vi "test_fastcast.vi"() -> ()   [LabVIEW 2013]
panel:
  out "data string":string
  out "default string":string[](array[string])
  out "default type":u8[](array[numeric]) format="%.0x"
  out "OK":bool[][](array[boolean])
  out "result":variant[][](array[variant])
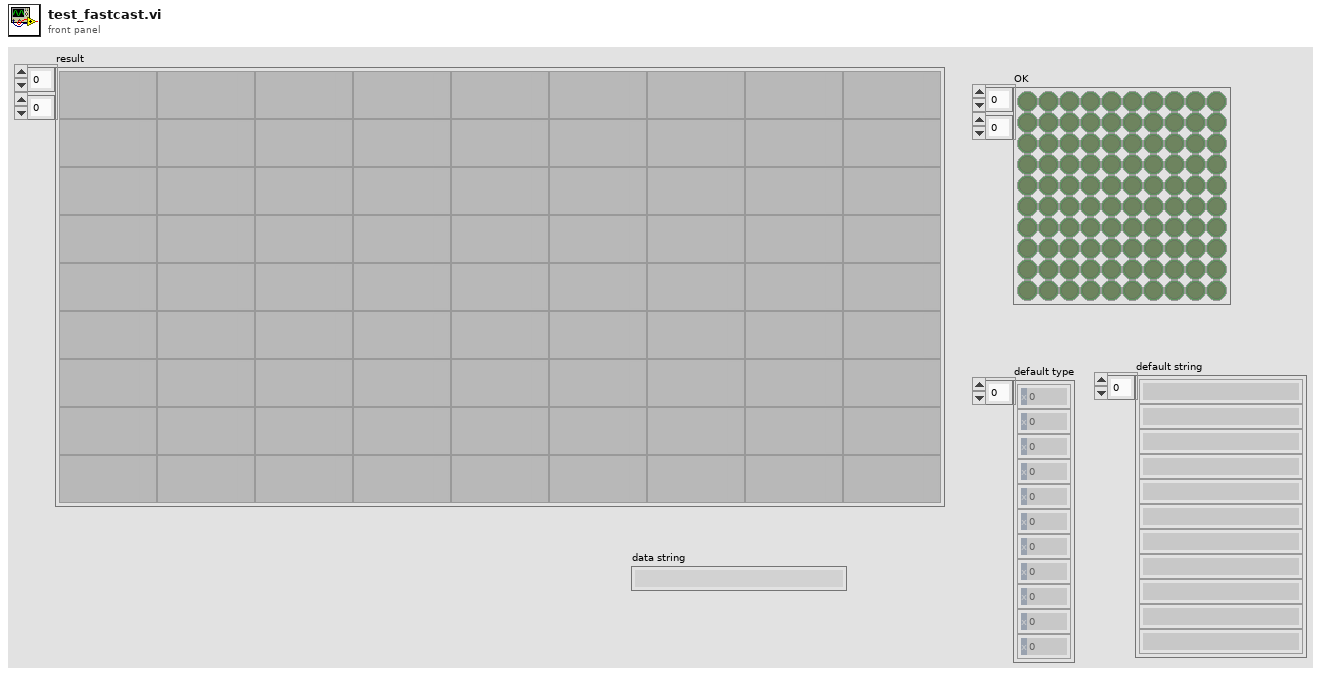
[diagram p1: front panel]
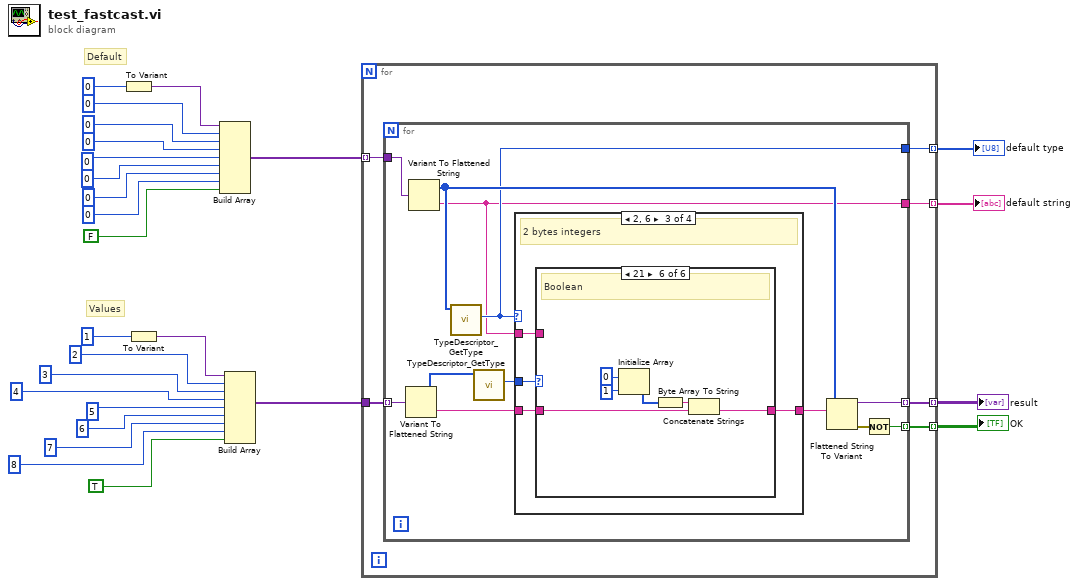
[diagram p0: block diagram]
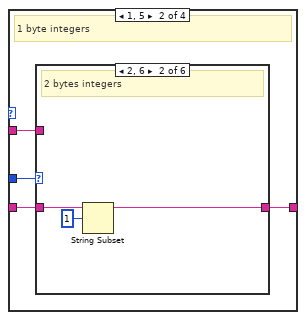
[diagram p3: hidden frame]
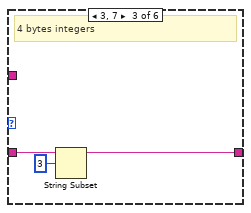
[diagram p5: hidden frame]
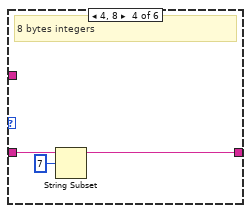
[diagram p6: hidden frame]
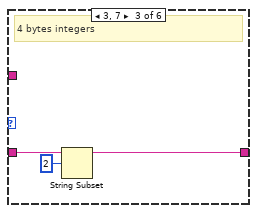
[diagram p11: hidden frame]
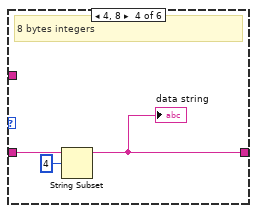
[diagram p12: hidden frame]
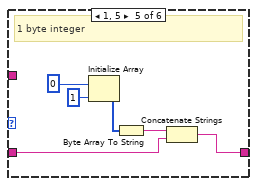
[diagram p13: hidden frame]
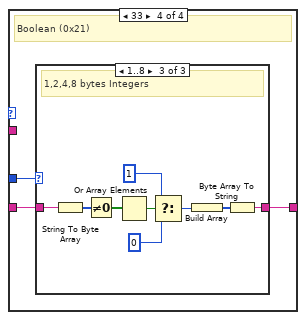
[diagram p14: hidden frame]
diagram:
  # "Values"
  # "Default"
  n1 = To Variant(anything=i8 0) -> (Variant=w25:variant)
  n2 = To Variant(anything=i8 1) -> (Variant=w2:variant)
  n3 = Build Array(w25, i16 0, 0, i64 0, u8 0, u16 0, u32 0, u64 0, FALSE) -> (w24:variant[])
  n4 = Build Array(w2, i16 2, 3, i64 4, u8 5, u16 6, u32 7, u64 8, TRUE) -> (w1:variant[])
  n5 = for {
    tunnel: w24 -> [w31] mode=indexing
    tunnel: w1 -> [w32]
    tunnel: [w30] -> w26 mode=indexing
    tunnel: [w29] -> w23 mode=indexing
    tunnel: [w28] -> w22 mode=indexing
    tunnel: [w27] -> w21 mode=indexing
    n6 = for {
      tunnel: w32 -> [w42] mode=indexing
      tunnel: w31 -> [w43]
      tunnel: [w41] -> w30 mode=indexing
      tunnel: [w44] -> w29 mode=indexing
      tunnel: [w34] -> w28
      tunnel: [w33] -> w27
      n7 = Variant To Flattened String(Variant=w42) -> (data string=w37:string, 1:w36:i16[])
      n8 = Variant To Flattened String(Variant=w43) -> (data string=w33:string, 1:w39:i16[])
      n9 = call "TypeDescriptor_GetType.vi"("type descriptor"=w39) -> ("Type"=w34:u8)  [unwired: 9 in, 1 out]
      n10 = call "TypeDescriptor_GetType.vi"("type descriptor"=w36) -> ("Type"=w35:u8)  [unwired: 9 in, 1 out]
      n11 = case shown="2, 6" w34 {
        tunnel: w37 -> [w45 w48 w63 w85]
        tunnel: [w45 w47 w62 w84] -> w38
        tunnel: w35 -> [_ w49 w64 w86]
        tunnel: w33 -> [_ w46 w61 _]
        frame Default {
        }
        frame 1, 5 {
          # "1 byte integers"
          n12 = case shown="2, 6" w49 {
            tunnel: w48 -> [_ w52 w55 w58 w59 w60]
            tunnel: [_ w50 w53 w56 w59 w60] -> w47
            tunnel: w46 -> [_ _ _ _ _ _]
            frame Default {
            }
            frame 2, 6 {
              # "2 bytes integers"
              n13 = String Subset(string=w52, offset (0)=1) -> (substring=w50:string)  [unwired: 1 in]
            }
            frame 3, 7 {
              # "4 bytes integers"
              n14 = String Subset(string=w55, offset (0)=3) -> (substring=w53:string)  [unwired: 1 in]
            }
            frame 4, 8 {
              # "8 bytes integers"
              n15 = String Subset(string=w58, offset (0)=7) -> (substring=w56:string)  [unwired: 1 in]
            }
            frame 1, 5 {
              # "1 bytesintegers"
            }
            frame 33 {
              # "Boolean"
            }
          }
        }
        frame 2, 6 {
          # "2 bytes integers"
          n16 = case shown="21" w64 {
            tunnel: w63 -> [_ w65 w68 w71 w73 w80]
            tunnel: [_ w65 w66 w69 w72 w79] -> w62
            tunnel: w61 -> [_ _ _ _ _ _]
            frame Default {
            }
            frame 2, 6 {
              # "2 bytes integers"
            }
            frame 3, 7 {
              # "4 bytes integers"
              n17 = String Subset(string=w68, offset (0)=2) -> (substring=w66:string)  [unwired: 1 in]
            }
            frame 4, 8 {
              # "8 bytes integers"
              n18 = String Subset(string=w71, offset (0)=4) -> (substring=w69:string)  [unwired: 1 in]
              "data string" <- w69
            }
            frame 1, 5 {
              # "1 byte integer"
              n19 = Initialize Array(u8 0, 1 ("dimension size")) -> (w75:u8[])
              n20 = Byte Array To String(unsigned byte array=w75) -> (string=w74:string)
              n21 = Concatenate Strings(w74, w73) -> (w72:string)
            }
            frame 33 {
              # "Boolean"
              n22 = Initialize Array(u8 0, 1 ("dimension size")) -> (w81:u8[])
              n23 = Byte Array To String(unsigned byte array=w81) -> (string=w78:string)
              n24 = Concatenate Strings(w78, w80) -> (w79:string)
            }
          }
        }
        frame 33 {
          # "Boolean (0x21)"
          n25 = case shown="1..8" w86 {
            tunnel: w85 -> [_ w87 w94]
            tunnel: [_ w87 w96] -> w84
            frame Default {
              # "Incompatible type"
            }
            frame 33 {
              # "Boolean (0x21)"
            }
            frame 1..8 {
              # "1,2,4,8 bytes Integers"
              n26 = String To Byte Array(string=w94) -> (unsigned byte array=w93:u8[])
              n27 = Not Equal To 0?(x=w93) -> (x != 0?=w92:bool[])
              n28 = Or Array Elements(Boolean array=w92) -> (logical OR=w91:bool)
              n29 = Select(t=u8 1, s=w91, f=u8 0) -> (s? t:f=w88:u8)
              n30 = Build Array(w88) -> (w95:u8[])
              n31 = Byte Array To String(unsigned byte array=w95) -> (string=w96:string)
            }
          }
        }
      }
      n32 = Flattened String To Variant(6:w38, 7:w39) -> (0:w40:errorcluster, 3:w41:variant)  [unwired: 1 in]
      n33 = Not(x=w40) -> (.not. x?=w44:bool)
    }
  }
  "result" <- w26
  "OK" <- w23
  "default type" <- w22
  "default string" <- w21
